vi "Servo MSMT Configure ET Timing Search Step.vi"(8 "error in (no error)":errorcluster, 11 "Servo MSMT in":refnum<class "Servo MSMT.lvclass">) -> (0 "error out":errorcluster, 3 "Servo MSMT out":refnum<class "Servo MSMT.lvclass">)   [LabVIEW 2014, in "Servo MSMT.lvclass"]
uses:
  Servo MSMT.lvclass
  QPA Measurement/QPA Measurement.lvlibp/Sequence Automation/Classes/QPA Measurement/QPA Measurement.lvclass
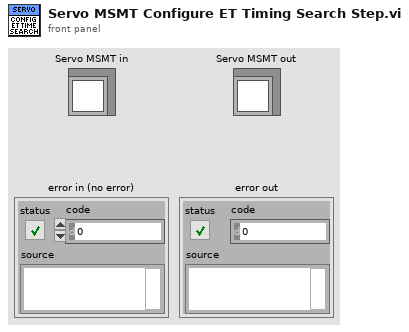
[diagram p1: front panel]
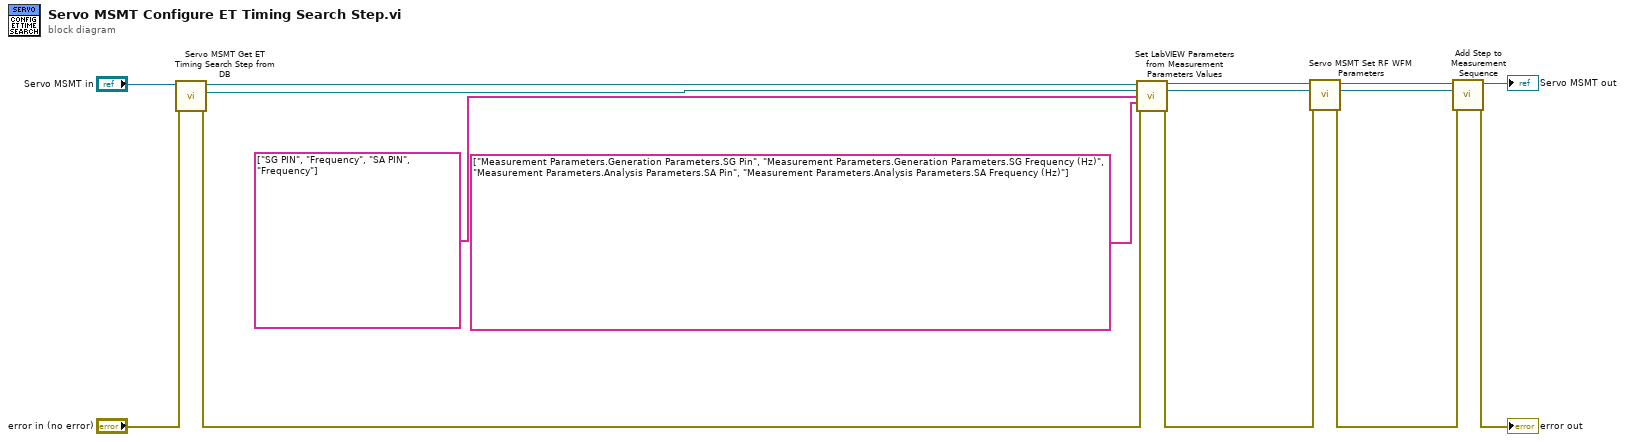
[diagram p0: block diagram]
diagram:
  n1 = call "Servo MSMT Get ET Timing Search Step from DB.vi"("error in (no error)"="error in (no error)", "Servo MSMT in"="Servo MSMT in") -> ("error out"=w7:errorcluster, "Step Out"=w8:refnum<k7>, "Servo MSMT out"=w9:refnum<class "Servo MSMT.lvclass">)  [unwired: 7 in]
  n2 = call "Set LabVIEW Parameters from Measurement Parameters Values.vi"("QPA Measurement in"=w9, "Step In"=w8, "Dictionary Keys"=string[] ["SG PIN", "Frequency", "SA PIN", "Frequency"] ("Database Keys"), "LabVIEW Parameter Mapping"=string[] ["Measurement Parameters.Generation Parameters.SG Pin", "Measurement Parameters.Generation Parameters.SG Frequency (Hz)", "Measurement Parameters.Analysis Parameters.SA Pin", "Measurement Parameters.Analysis Parameters.SA Frequency (Hz)"] ("Database Keys"), "error in (no error)"=w7) -> ("QPA Measurement out"=w4:refnum<class "Servo MSMT.lvclass">, "Step Out"=w3:refnum<k7>, "error out"=w6:errorcluster)  [unwired: 8 in]
  n3 = call "Servo MSMT Set RF WFM Parameters.vi"("error in (no error)"=w6, "Step In"=w3, "Servo MSMT in"=w4) -> ("error out"=w5:errorcluster, "Step Out"=w1:refnum<k7>, "Servo MSMT out"=w2:refnum<class "Servo MSMT.lvclass">)  [unwired: 6 in]
  n4 = call "Add Step to Measurement Sequence.vi"("error in (no error)"=w5, "Step to Add"=w1, "QPA Measurement in"=w2) -> ("error out"=→"error out":errorcluster, "QPA Measurement out"=→"Servo MSMT out":refnum<class "Servo MSMT.lvclass">)  [unwired: 7 in]
